vi "BT DUT Additional Defaults.vi"(0 "niDTS BT DUT in":refnum<class "niDTS BT Dut.lvclass">, 11 "error in (no error)":errorcluster) -> (4 "niDTS BT DUT out":refnum<class "niDTS BT Dut.lvclass">, 15 "error out":errorcluster)   [LabVIEW 2015, in "niDTS BT.lvlib" / "niDTS BT Dut.lvclass"]
doc: "This allows additional defaults to be set after the primary parameters (Standard, Rate, Bandwidth, Streams) have been set. The base additionally sets FEC Coding (BCC for HT and LDPC for VHT) and 16 symbols to True. This can be overridden by specific DUT controllers to impliment the desired behavior."
uses:
  niDTS BT Dut.lvclass
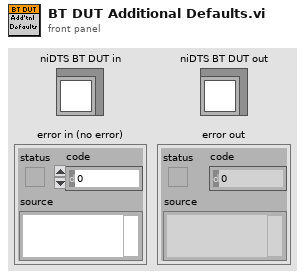
[diagram p1: front panel]
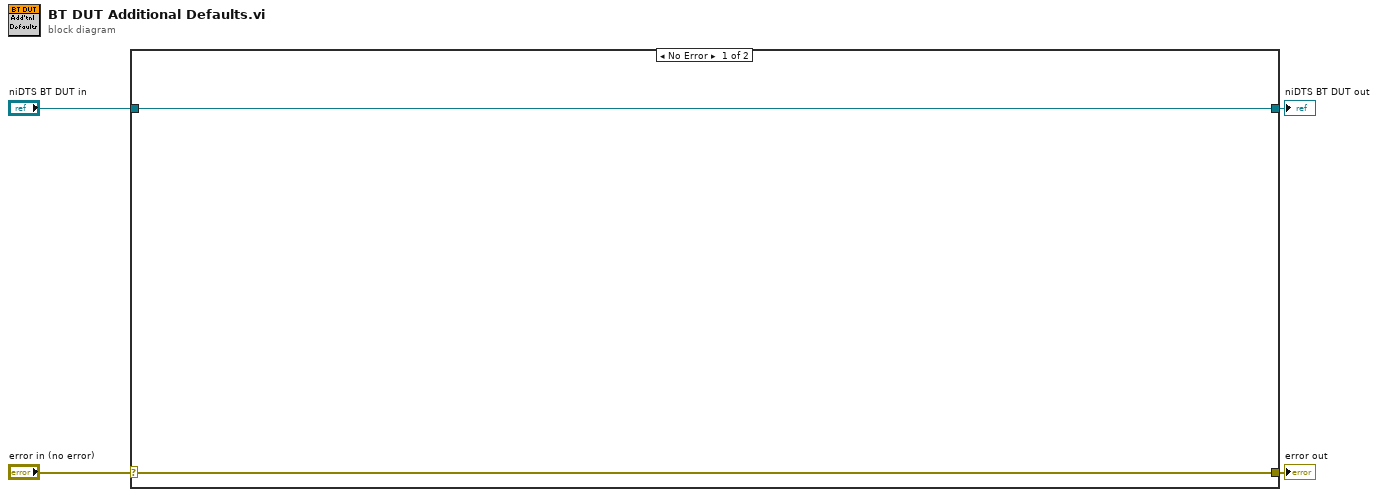
[diagram p0: block diagram]
diagram:
  n1 = case shown="No Error" "error in (no error)" {
    selector: "error in (no error)" -> [w6 w8]
    tunnel: [w6 w8] -> w3
    tunnel: [w5 w7] -> w1
    tunnel: "niDTS BT DUT in" -> [w5 w7]
    frame No Error {
    }
    frame Error {
    }
  }
  "error out" <- w3
  "niDTS BT DUT out" <- w1
